vi "CheckEndDCS.vi"(0 "start":bool=TRUE, 7 "duration time":sgl=2500.0, 11 "elapsed time":sgl=2500.0) -> (6 "stopped":bool, 10 "time left":sgl format="%.3f")   [LabVIEW 2011]
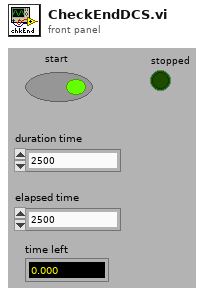
[diagram p1: front panel]
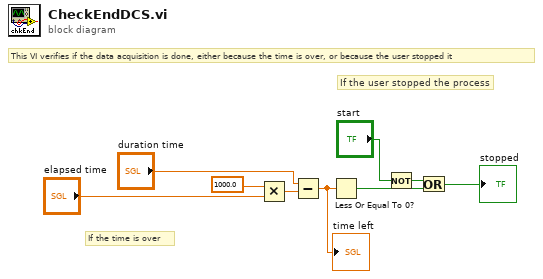
[diagram p0: block diagram]
diagram:
  # "This VI verifies if the data acquisition is done, either because the time is over, or because the user stopped it"
  # "If the time is over"
  # "If the user stopped the process"
  n1 = Multiply(x=sgl 1000.0, y="elapsed time") -> (x*y=w8:sgl)
  n2 = Subtract(x="duration time", y=w8) -> (x-y=w6:sgl)
  "time left" <- w6
  n3 = Less Or Equal To 0?(x=w6) -> (x <= 0?=w7:bool)
  n4 = Not(x="start") -> (.not. x?=w3:bool)
  n5 = Or(x=w3, y=w7) -> (x .or. y?=→"stopped":bool)
